vi "S2C_FORNAX_Proc_MessageFGV.vi"(7 "Action":enum16{"Set", "Get"}(ring), 8 "Error In":errorcluster, 11 "Msg In":T1) -> (0 "Error Out":errorcluster, 3 "Msg Out":T1)   [LabVIEW 2015]
doc: "Keeps the ViperMsg and DDSMsg arrays to 1000 characters or less."
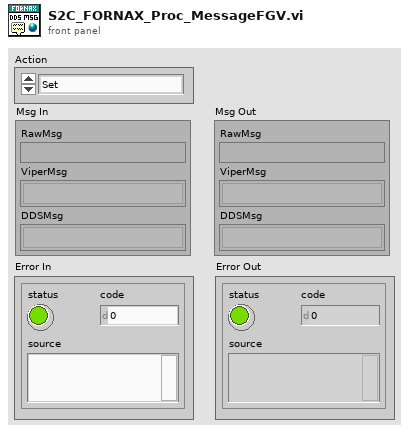
[diagram p1: front panel]
types:
  T1 = cluster{"RawMsg":string, "ViperMsg":string[], "DDSMsg":string[]}
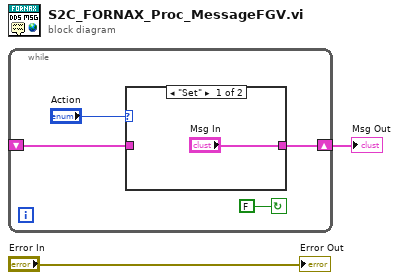
[diagram p0: block diagram]
diagram:
  n1 = while {
    shift-right: [w4] -> w1
    shift-left: _ -> [w3]
    stop <- FALSE continue-if-true
    n2 = case shown="\"Set\"" "Action" {
      tunnel: ["Msg In" w8] -> w4
      tunnel: w3 -> [_ w8]
      frame "Set" {
      }
      frame "Get" {
      }
    }
  }
  "Msg Out" <- w1
  "Error Out" <- "Error In"
